vi "FFT滤波模块.vi"() -> ()   [LabVIEW 2014]
uses:
  <vilib>/Analysis/3filter.llb/Filter Passband Type.ctl
  <vilib>/Analysis/2dsp.llb/Real FFT.vi
  <vilib>/Analysis/2dsp.llb/Inverse Real FFT.vi
  <vilib>/measure/maspectr.llb/FFT Spectrum (Mag-Phase) for 1 Chan.vi
  <vilib>/Analysis/3filter.llb/Butterworth Filter (CDB).vi
  <vilib>/Analysis/NI_AALPro.lvlib
  <vilib>/Analysis/NI_AALBase.lvlib
  <vilib>/measure/NI_MABase.lvlib
  <vilib>/measure/NI_MAPro.lvlib
panel:
  out "时域波形图 4":cluster{"f0":dbl, "df":dbl, "magnitude":dbl[]}(graph)
  out "时域波形图 3":waveform(dbl)(graph)
  out "时域波形图 2":waveform(dbl)(graph)
  in  "low cutoff freq: fl":dbl=0.12500000000000006 caption="低截止频率:fl" format="%0.4f"
  in  "sampling freq: fs":dbl=1.0 caption="采样频率:fs" format="%0.2f"
  in  "时域波形图":waveform(dbl)[](graph)
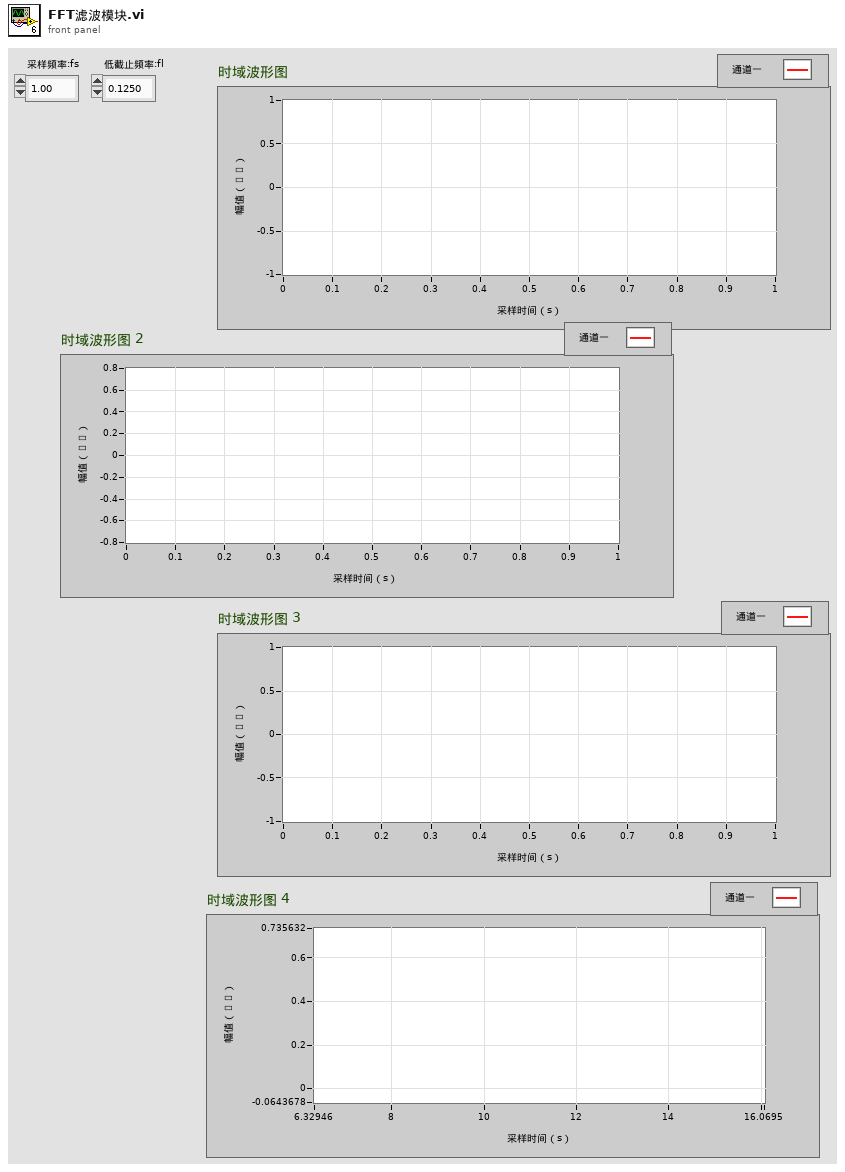
[diagram p1: front panel]
types:
  T1 = typedef "NI_AALBase.lvlib/Filter Passband Type.ctl" = enum32{"Lowpass", "Highpass", "Bandpass", "Bandstop"}
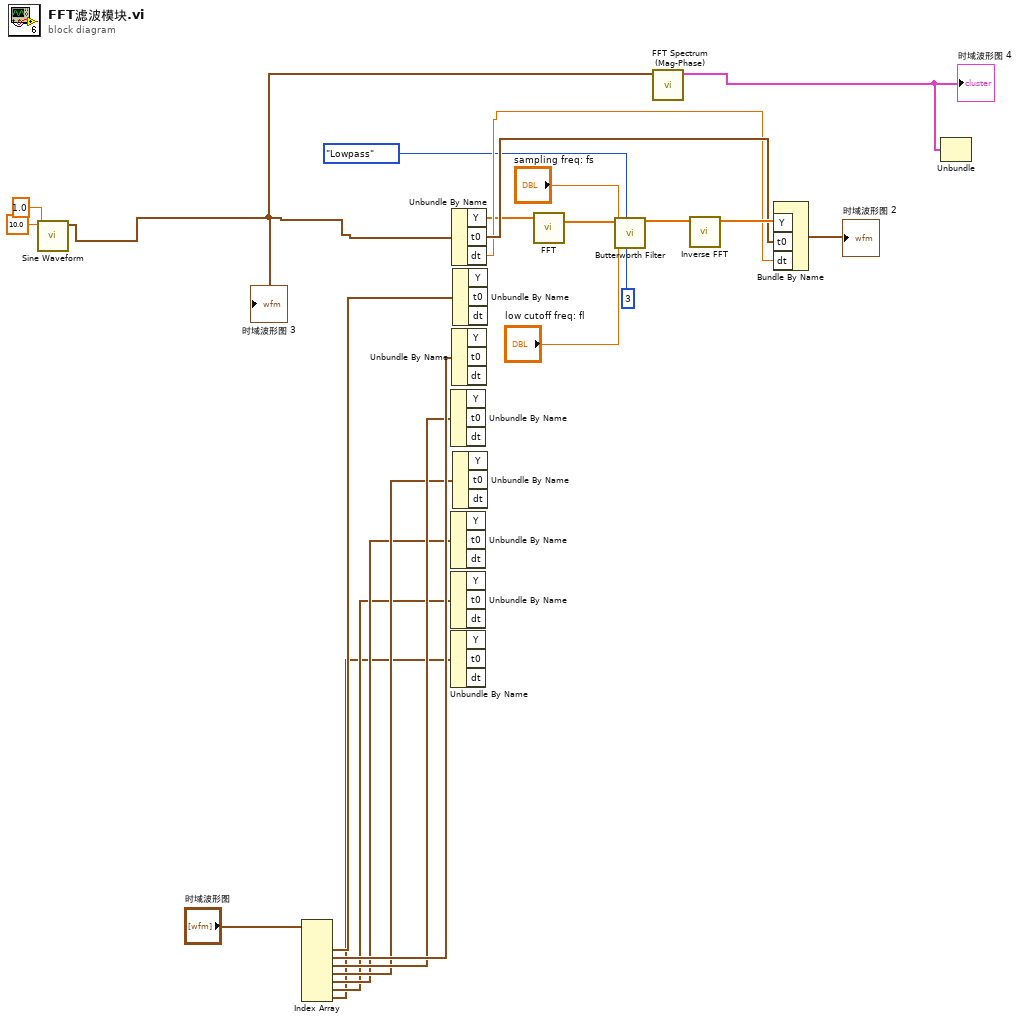
[diagram p0: block diagram]
diagram:
  n1 = call <vilib>:"Sine Waveform.vi"("amplitude"=1.0, "frequency"=10.0) -> ("signal out"=w2:waveform(dbl))  [unwired: 8 in, 1 out]
  "时域波形图 3" <- w2
  n2 = Index Array(array="时域波形图") -> (element #2=w22:waveform(dbl), element #3=w21:waveform(dbl), element #4=w20:waveform(dbl), element #5=w19:waveform(dbl), element #6=w18:waveform(dbl), element #7=w17:waveform(dbl), element #8=w16:waveform(dbl))  [unwired: 8 in, 1 out]
  n3 = Unbundle By Name(w20) -> ()  [unwired: 3 out]
  n4 = Unbundle By Name(w18) -> ()  [unwired: 3 out]
  n5 = Unbundle By Name(w17) -> ()  [unwired: 3 out]
  n6 = Unbundle By Name(w16) -> ()  [unwired: 3 out]
  n7 = Unbundle By Name(w2) -> ("Y"=w4:dbl[], "t0"=w11:timestamp, "dt"=w10:dbl)
  n8 = Unbundle By Name(w21) -> ()  [unwired: 3 out]
  n9 = Unbundle By Name(w22) -> ()  [unwired: 3 out]
  n10 = Unbundle By Name(w19) -> ()  [unwired: 3 out]
  n11 = call-poly <vilib>:"FFT.vi"("X"=w4) -> ("FFT {X}"=w3:cdb[])  [unwired: 9 in, 1 out]
  n12 = call-poly <vilib>:"Butterworth Filter.vi"("order"=3, "filter type"=Filter_Passband_Type."Lowpass", "low cutoff freq: fl"="low cutoff freq: fl", "sampling freq: fs"="sampling freq: fs", "X"=w3) -> ("Filtered X"=w13:cdb[])  [unwired: 3 in, 1 out]
  n13 = call-poly <vilib>:"FFT Spectrum (Mag-Phase).vi"("time signal"=w2) -> ("magnitude"=w1:cluster{"f0":dbl, "df":dbl, "magnitude":dbl[]})  [unwired: 6 in, 4 out]
  "时域波形图 4" <- w1
  n14 = call-poly <vilib>:"Inverse FFT.vi"("FFT {X}"=w13) -> ("X"=w12:dbl[])  [unwired: 9 in, 1 out]
  n15 = Bundle By Name("Y"=w12, "t0"=w11, "dt"=w10) -> (→"时域波形图 2":waveform(dbl))  [unwired: 1 in]
  n16 = Unbundle(w1) -> ()  [unwired: 3 out]
